vi "Begin.vi"(8 "error in (no error)":errorcluster, 9 "Left":T1, 10 "Right":T1, 11 "Simulated Drive in":refnum<class "Simulated Drive.lvclass">) -> (0 "error out":errorcluster, 3 "Simulated Drive out":refnum<class "Simulated Drive.lvclass">)   [LabVIEW 2018, in "Drive.lvlib" / "Simulated Drive.lvclass"]
doc: "This VI holds the begin code"
uses:
  Simulated Drive.lvclass
  Pod Drive/Pod.ctl
  Drive.lvclass
  Pod Drive/Pod Drive.lvclass
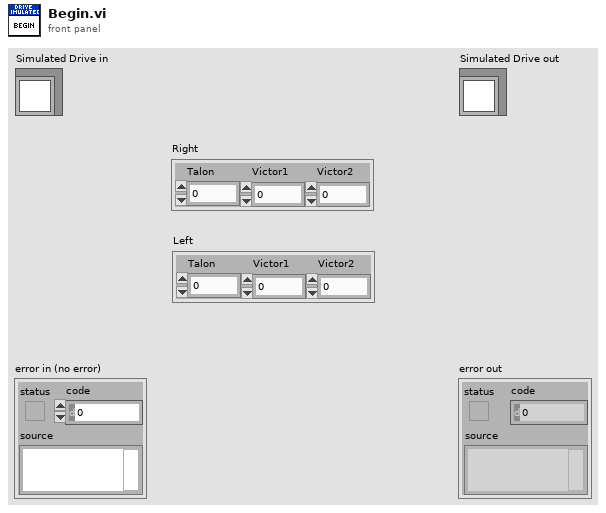
[diagram p1: front panel]
types:
  T1 = typedef "Drive.lvlib/Pod Drive.lvclass/Pod.ctl" = cluster{"Talon":u8, "Victor1":u8, "Victor2":u8}
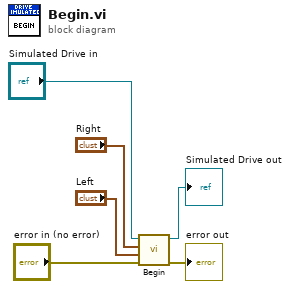
[diagram p0: block diagram]
diagram:
  n1 = call-parent "Begin.vi"("error in (no error)"="error in (no error)", "Left"="Left", "Right"="Right", "Drive in"="Simulated Drive in") -> ("error out"=→"error out":errorcluster, "Drive out"=→"Simulated Drive out":refnum<class "Simulated Drive.lvclass">)  [unwired: 6 in]
